vi "Library - By Folder.vi"(7 "Msg Chain":string, 8 "error in (no error)":errorcluster {"code" format="Error %.0f"}, 10 "Libraries":refnum<class "Library Documentation.lvclass">[](array[class]), 11 "VIDoc Printer - Confluence In":refnum<class "VIDoc Printer - Confluence.lvclass">) -> (0 "error out":errorcluster {"code" format="Error %.0f"}, 3 "VIDoc Printer - Confluence Out":refnum<class "VIDoc Printer - Confluence.lvclass">)   [LabVIEW 2023, in "VIDoc Printer - Confluence.lvlib" / "VIDoc Printer - Confluence.lvclass"]
uses:
  VIDoc Printer - Confluence.lvclass
  Parsing/Library Documentation/Library Documentation.lvclass
  Confluence Formatting/Types/Format Combo Box.ctl
  VIDoc Printer - Confluence.lvclass/VIDoc Printer - Confluence.ctl
  Parsing/Library Documentation/Library Documentation.lvclass/Library Documentation.ctl
  Parsing/Library Documentation/Get Path.vi
  Accessors/Get Library By Folder Expand.vi
  Confluence Formatting/Confluence Formatting.lvlib
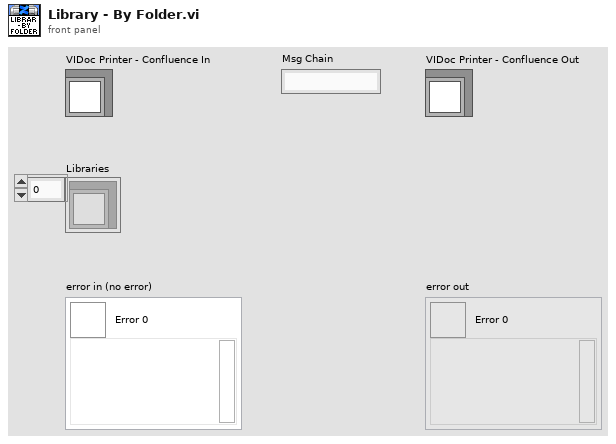
[diagram p1: front panel]
types:
  T1 = typedef "Confluence Formatting.lvlib/Format Combo Box.ctl" = string
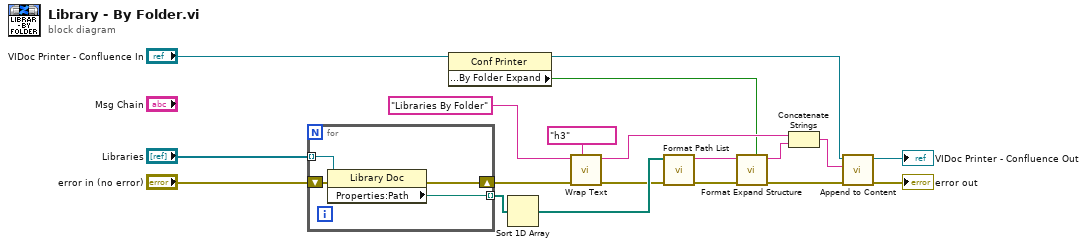
[diagram p0: block diagram]
diagram:
  n1 = for {
    tunnel: "Libraries" -> [w22] mode=indexing
    tunnel: [w20] -> w18 mode=indexing
    shift-right: [w21] -> w17
    shift-left: "error in (no error)" -> [w23]
    n2 = property class="Library Doc"(reference=w22, error in=w23) -> (error out=w21:errorcluster, "Properties:Path"=w20:path)  [unwired: 1 out]
  }
  n3 = property class="Conf Printer"(reference="VIDoc Printer - Confluence In") -> (reference out=w2:refnum<class "VIDoc Printer - Confluence.lvclass">, "Properties:Expand?:Library:By Folder Expand"=w1:bool)  [unwired: 1 in, 1 out]
  n4 = Sort 1D Array(array=w18) -> (sorted array=w14:path[])
  n5 = call "Wrap Text.vi"("Formatting"=T1 "h3", "Error in"=w17, "String"="Libraries By Folder") -> ("Error out"=w13:errorcluster, "Wrapped String"=w16:string)  [unwired: 7 in]
  n6 = call "Format Path List.vi"("Error in"=w13, "Paths"=w14) -> ("Error out"=w12:errorcluster, "Bullet List String"=w4:string)  [unwired: 8 in]
  n7 = call "Format Expand Structure.vi"("Enable? (T)"=w1, "Error in"=w12, "Content"=w4) -> ("Error out"=w5:errorcluster, "Expand String"=w3:string)  [unwired: 7 in]
  n8 = Concatenate Strings(w16, w3) -> (w15:string)
  n9 = call "Append to Content.vi"("error in (no error)"=w5, "Content"=w15, "VIDoc Printer - Confluence In"=w2) -> ("error out"=→"error out":errorcluster, "VIDoc Printer - Confluence Out"=→"VIDoc Printer - Confluence Out":refnum<class "VIDoc Printer - Confluence.lvclass">)  [unwired: 7 in]
